vi "Configure Temperature (Thermocouple).vi"(0 "VISA resource name":refnum<visa-resource-name>, 1 "Reference Junction Temperature (10)":dbl=10.0, 5 "Thermocouple Type (0: B Type)":u16(ring) items=["B Type", "E Type", "J Type", "K Type", "N Type", "R Type", "S Type", "T Type"], 7 "Reference Junction Type (0: Fixed Value)":u16(ring) items=["Fixed Value", "Internal Thermistor", "External Thermistor"], 9 "Units (0: Celsius)":u16(ring) items=["Celsius", "Fahrenheit", "Kelvin"], 11 "error in (no error)":errorcluster) -> (4 "VISA resource name out":refnum<visa-resource-name>, 15 "error out":errorcluster)   [LabVIEW 2021, in "Agilent 34420.lvlib"]
doc: "Configures the thermocouple settings for temperature measurements."
uses:
  <instrlib>/Agilent 34420/Agilent 34420.lvlib
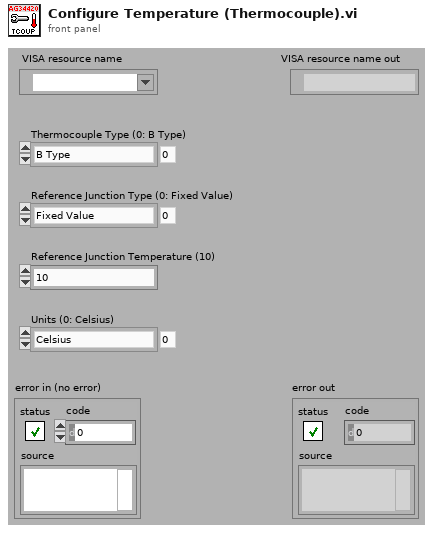
[diagram p1: front panel]
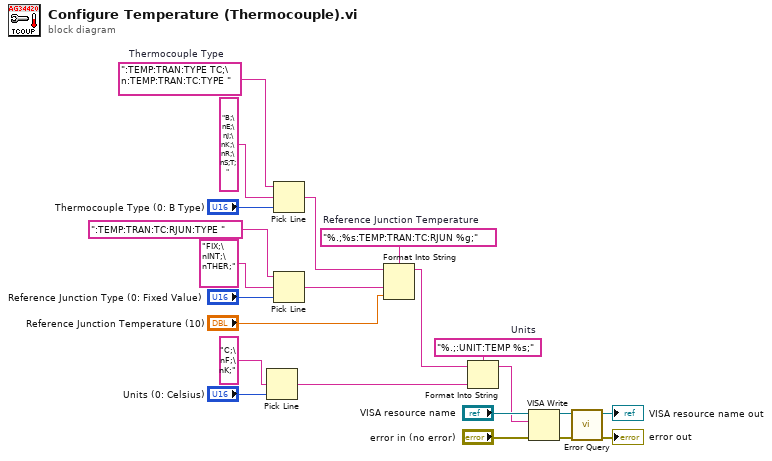
[diagram p0: block diagram]
diagram:
  w3 = "%.;:UNIT:TEMP %s;"  # Units
  w7 = "%.;%s:TEMP:TRAN:TC:RJUN %g;"  # Reference Junction Temperature
  w13 = ":TEMP:TRAN:TYPE TC;\n:TEMP:TRAN:TC:TYPE "  # Thermocouple Type
  n1 = Pick Line(multi-line string="C;\nF;\nK;", line index="Units (0: Celsius)") -> (output string=w4:string)  [unwired: 1 in]
  n2 = Pick Line(string ("")=w13, multi-line string="B;\nE;\nJ;\nK;\nR;\nS;T;", line index="Thermocouple Type (0: B Type)") -> (output string=w10:string)
  n3 = Pick Line(string ("")=":TEMP:TRAN:TC:RJUN:TYPE ", multi-line string="FIX;\nINT;\nTHER;" ("Ref Junction Type"), line index="Reference Junction Type (0: Fixed Value)") -> (output string=w9:string)
  n4 = Format Into String(format string=w7, initial string=w10, w9, "Reference Junction Temperature (10)") -> (resulting string=w1:string)  [unwired: 1 in, 1 out]
  n5 = Format Into String(format string=w3, initial string=w1, w4) -> (resulting string=w2:string)  [unwired: 1 in, 1 out]
  n6 = VISA Write(VISA resource name="VISA resource name", write buffer=w2, error in (no error)="error in (no error)") -> (VISA resource name out=w16:refnum<visa-resource-name>, error out=w15:errorcluster)  [unwired: 1 out]
  n7 = call <instrlib>:"Error Query.vi"("error in (no error)"=w15, "VISA resource name"=w16) -> ("error out"=→"error out":errorcluster, "VISA resource name out"=→"VISA resource name out":refnum<visa-resource-name>)  [unwired: 6 in, 2 out]
